vi "set_up_2700.vi"(8 "Serial Configuration":T1, 11 "VISA Refnum in":refnum<visa-resource-name>) -> (0 "error out":errorcluster, 3 "VISA Refnum out":refnum<visa-resource-name>)   [LabVIEW 2011]
uses:
  <instrlib>/Keithley 27XX/Public/Configure/Measurement Specific/Configure FRTD.vi
  <instrlib>/Keithley 27XX/Keithley 27XX.lvlib
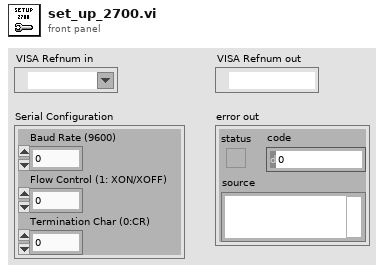
[diagram p1: front panel]
types:
  T1 = cluster{"Baud Rate (9600)":u32, "Flow Control (1: XON/XOFF)":u16, "Termination Char (0:CR)":u16}
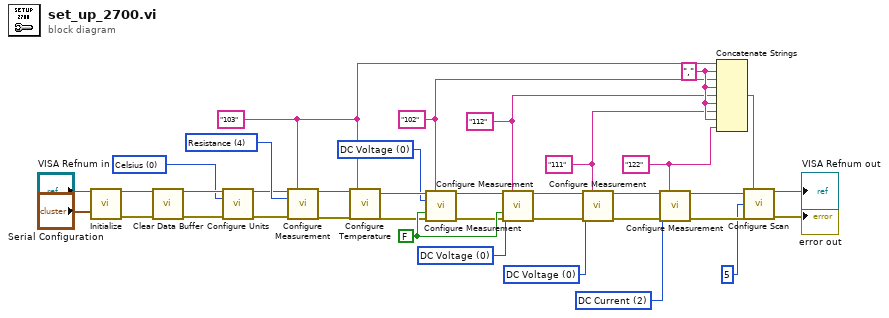
[diagram p0: block diagram]
diagram:
  w35 = u16 2 items=["DC Voltage", "AC Voltage", "DC Current", "AC Current", "Resistance", "Four-Wire Resistance", "Temperature", "Frequency", "Period", "Continuity"] ("Function (0: DC Voltage)")
  w36 = "122" ("Scan List (Empty)")
  w30 = FALSE ("Enable Auto Range (True)")
  w29 = "111" ("Scan List (Empty)")
  w28 = u16 0 items=["DC Voltage", "AC Voltage", "DC Current", "AC Current", "Resistance", "Four-Wire Resistance", "Temperature", "Frequency", "Period", "Continuity"] ("Function (0: DC Voltage)")
  w23 = u16 0 items=["DC Voltage", "AC Voltage", "DC Current", "AC Current", "Resistance", "Four-Wire Resistance", "Temperature", "Frequency", "Period", "Continuity"] ("Function (0: DC Voltage)")
  w37 = "," ("string")
  w19 = "103"
  w24 = "112" ("Scan List (Empty)")
  w25 = "102" ("Scan List (Empty)")
  w16 = u16 0 items=["DC Voltage", "AC Voltage", "DC Current", "AC Current", "Resistance", "Four-Wire Resistance", "Temperature", "Frequency", "Period", "Continuity"] ("Function (0: DC Voltage)")
  w5 = u16 0 items=["Celsius", "Fahrenheit", "Kelvin"] ("Temperature (0: Celsius)")
  w3 = u16 4 items=["DC Voltage", "AC Voltage", "DC Current", "AC Current", "Resistance", "Four-Wire Resistance", "Temperature (C)", "Frequency", "Period", "Continuity"] ("Function (0: DC Voltage)")
  n1 = call <instrlib>:"Initialize.vi"("VISA resource name"="VISA Refnum in", "Serial Configuration"="Serial Configuration") -> ("VISA resource name out"=w12:refnum<visa-resource-name>, "error out"=w14:errorcluster)  [unwired: 12 in]
  n2 = call <instrlib>:"Clear Data Buffer.vi"("VISA resource name"=w12, "error in (no error)"=w14) -> ("VISA resource name out"=w13:refnum<visa-resource-name>, "error out"=w15:errorcluster)  [unwired: 12 in]
  n3 = call <instrlib>:"Configure Units.vi"("VISA resource name"=w13, "Temperature (0: Celsius)"=w5, "error in (no error)"=w15) -> ("VISA resource name out"=w2:refnum<visa-resource-name>, "error out"=w8:errorcluster)  [unwired: 11 in]
  n4 = call <instrlib>:"Configure Measurement.vi"("VISA resource name"=w2, "Scan List (Empty)"=w19, "Function (0: DC Voltage)"=w3, "error in (no error)"=w8) -> ("VISA resource name out"=w9:refnum<visa-resource-name>, "error out"=w1:errorcluster)  [unwired: 10 in]
  n5 = call-poly <instrlib>:"Configure Temperature.vi"("VISA resource name"=w9, "error in (no error)"=w1, "Scan List (Empty)"=w19) -> ("VISA resource name out"=w17:refnum<visa-resource-name>, "error out"=w18:errorcluster)  [unwired: 15 in]
  n6 = call <instrlib>:"Configure Measurement.vi"("VISA resource name"=w17, "Scan List (Empty)"=w25, "Function (0: DC Voltage)"=w16, "Enable Auto Range (True)"=w30, "error in (no error)"=w18) -> ("VISA resource name out"=w21:refnum<visa-resource-name>, "error out"=w22:errorcluster)  [unwired: 9 in]
  n7 = call <instrlib>:"Configure Measurement.vi"("VISA resource name"=w21, "Scan List (Empty)"=w24, "Function (0: DC Voltage)"=w23, "Enable Auto Range (True)"=w30, "error in (no error)"=w22) -> ("VISA resource name out"=w26:refnum<visa-resource-name>, "error out"=w27:errorcluster)  [unwired: 9 in]
  n8 = call <instrlib>:"Configure Measurement.vi"("VISA resource name"=w26, "Scan List (Empty)"=w29, "Function (0: DC Voltage)"=w28, "error in (no error)"=w27) -> ("VISA resource name out"=w31:refnum<visa-resource-name>, "error out"=w33:errorcluster)  [unwired: 10 in]
  n9 = call <instrlib>:"Configure Measurement.vi"("VISA resource name"=w31, "Scan List (Empty)"=w36, "Function (0: DC Voltage)"=w35, "error in (no error)"=w33) -> ("VISA resource name out"=w32:refnum<visa-resource-name>, "error out"=w34:errorcluster)  [unwired: 10 in]
  n10 = Concatenate Strings(w19, w37, w25, w37, w24, w37, w29, w37, w36) -> (w20:string)
  n11 = call <instrlib>:"Configure Scan.vi"("VISA resource name"=w32, "Channel List (101:110)"=w20, "Sample Count (100)"=5, "error in (no error)"=w34) -> ("VISA resource name out"=→"VISA Refnum out":refnum<visa-resource-name>, "error out"=→"error out":errorcluster)  [unwired: 10 in]
